vi "setBitS0_32.vi"(8 "error in (no error)":errorcluster, 9 "Address":u8, 10 "bitnumber":u32) -> (0 "error out":errorcluster)   [LabVIEW 2015, in "ESLSCDLL.lvlib"]
uses:
  ESLSCDLL.lvlib
  Globals.vi
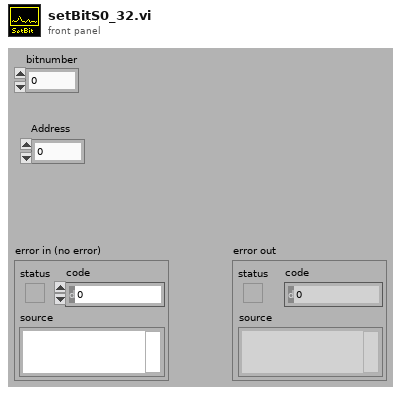
[diagram p1: front panel]
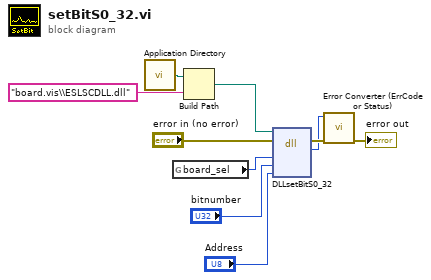
[diagram p0: block diagram]
diagram:
  n1 = call <vilib>:"Application Directory.vi"() -> ("Application Directory"=w4:path)
  n2 = global read "Globals.vi" "board_sel"() -> (w1:u32)
  n3 = Build Path(base path=w4, name or relative path="board.vis\\ESLSCDLL.dll") -> (appended path=w2:path)
  n4 = dll-call lib="C:/ENTW/PCIE/LV64/board.vis/ESLSCDLL.dll" fn="DLLsetBitS0_32" ("lwlscdll.dll:DLLRsTOREG")(path in=w2, error in="error in (no error)", "board_sel"=w1, "bitnumber"="bitnumber", "Address"="Address") -> (error out=w6:errorcluster, "es_status_codes"=w5:i32)  [unwired: 4 in, 1 out]
  n5 = call "Error Converter (ErrCode or Status).vi"("error in (no error)"=w6, "error code"=w5) -> ("error out"=→"error out":errorcluster)  [unwired: 9 in]
